vi "Run_NS3.vi"(8 "error in":errorcluster) -> (0 "error out":errorcluster, 1 "standard error":string, 3 "Performance":dbl)   [LabVIEW 2010]
doc: "This routine implements the execution of the NS3 scriipt and delivers the reuslts.\n\nCreated by Davis Montenegro\n06-27-2017"
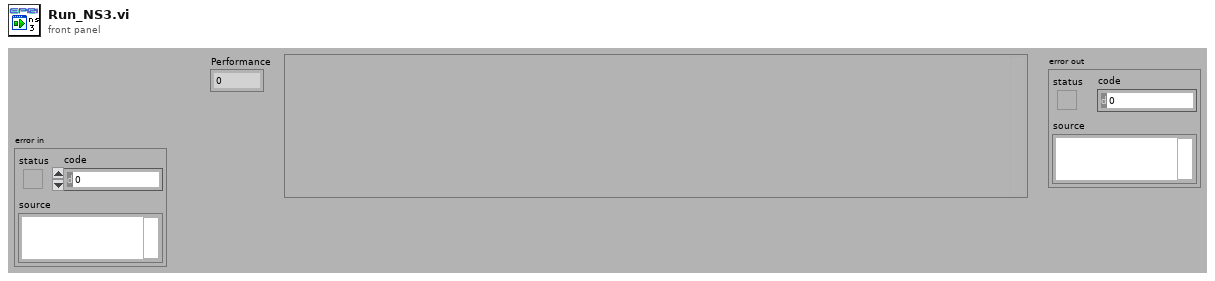
[diagram p1: front panel]
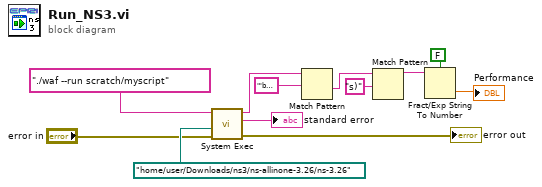
[diagram p0: block diagram]
diagram:
  n1 = call <vilib>:"System Exec.vi"("error in (no error)"="error in", "working directory"=path "/home/user/Downloads/ns3/ns-allinone-3.26/ns-3.26", "command line"="./waf --run scratch/myscript") -> ("error out"=→"error out":errorcluster, "standard error"=→"standard error":string, "standard output"=w5:string)  [unwired: 5 in, 1 out]
  n2 = Match Pattern(string=w5, regular expression="'build' finished successfully (") -> (after substring=w7:string)  [unwired: 1 in, 3 out]
  n3 = Match Pattern(string=w7, regular expression="s)") -> (before substring=w9:string)  [unwired: 1 in, 3 out]
  n4 = Fract/Exp String To Number(use system decimal point (T)=FALSE, string=w9) -> (number=→"Performance":dbl)  [unwired: 2 in, 1 out]
